vi "PH_IEEE1394Camera.set Cam Attribute GUI Elements for the first Time.vi"(0 "i ref in":refnum<vi>, 5 "error in (no error)":errorcluster) -> (14 "i ref out":refnum<vi>, 19 "error out":errorcluster)   [LabVIEW 2014, in "PH_IEEE1394Camera.lvlib"]
doc: "This VI gets several cam trigger attributes, sets them to own attributes and the GUI elements."
uses:
  PH_IEEE1394Camera.lvlib
  PH_Basics/PH_Common/PH_Common.lvlib
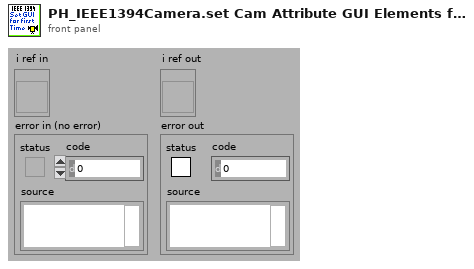
[diagram p1: front panel]
types:
  T1 = typedef "PH_IEEE1394Camera.lvlib/PH_IEEE1394Camera.i attribute.ctl" = cluster{"Gui Refs":cluster{"Brightness":refnum<vi>, "Shutter":refnum<vi>, "Gain":refnum<vi>, "Center of Gravity":refnum<vi>, "Supported Video Modes":refnum<vi>, "Trigger Polarity":refnum<vi>, "Trigger Mode":refnum<vi>, "Trigger Timeout":refnum<vi>, "Bit Depth":refnum<vi>, "Video Mode":refnum<vi>, "Top":refnum<vi>, "Bottom":refnum<vi>, "Left":refnum<vi>, "Right":refnum<vi>, "Set ROI to Maximum":refnum<vi>, "Camera Details":refnum<vi>, "Current Cam Attributes":refnum<vi>, "Attribute to set":refnum<vi>, "Num Value":refnum<vi>, "String Value":refnum<vi>, "Bool Value":refnum<vi>, "Set Cam Attribute":refnum<vi>}, "Cam":cluster{"IMAQ1394 Session":T2, "Camera Details":T3}, "Current Attributes":T4[], "Supported Video Modes ":cluster{"Video Mode":u32, "Video Mode Name":string}[], "Wanted Attributes":cluster{"Name":string, "Num Value":dbl, "String Value":string, "Boolean Value":bool}[], "Cam Attributes":T6}
  T2 = typedef "IMAQdx.ctl" = refnum<k21>
  T3 = typedef "PH_IEEE1394Camera.lvlib/PH_IEEE1394Camera.Cam Details.ctl" = cluster{"Model":string, "Serial Number":dbl, "Cam name (Machinery)":string, "Bus Type":string}
  T4 = typedef "PH_IEEE1394Camera.lvlib/PH_IEEE1394Camera.Cam Attribute.ctl" = cluster{"Information":cluster{"Type":T5, "Readable":bool, "Writable":bool, "Name":string}, "Num Value":dbl, "String Value":string, "Maximum":dbl, "Minimum":dbl, "Units":string, "Description":string, "EnumStrings[]":string[], "EnumValues[]":u32[], "Boolean Value":bool}
  T5 = typedef "NI_Vision_Acquisition_Software.lvlib/IMAQdx Attribute Type.ctl" = enum32{"U32", "I64", "DBL", "String", "Enum", "Bool", "Command"}
  T6 = typedef "PH_IEEE1394Camera.lvlib/PH_IEEE1394Camera.Relevant Cam Attributes.ctl" = cluster{"Video Mode":cluster{"Name":string, "Index":i32}, "Brightness":cluster{"Name":string, "Index":i32}, "Gain":cluster{"Name":string, "Index":i32}, "Shutter":cluster{"Name":string, "Index":i32}, "Trigger Pol":cluster{"Name":string, "Index":i32}, "Trigger Mode":cluster{"Name":string, "Index":i32}, "Timeout":cluster{"Name":string, "Index":i32}, "Bit Depth":cluster{"Name":string, "Index":i32}, "Pixel Bits":cluster{"Name":string, "Index":i32}, "Pixel Bytes":cluster{"Name":string, "Index":i32}, "Left":cluster{"Name":string, "Index":i32}, "Right":cluster{"Name":string, "Index":i32}, "Top":cluster{"Name":string, "Index":i32}, "Bottom":cluster{"Name":string, "Index":i32}}
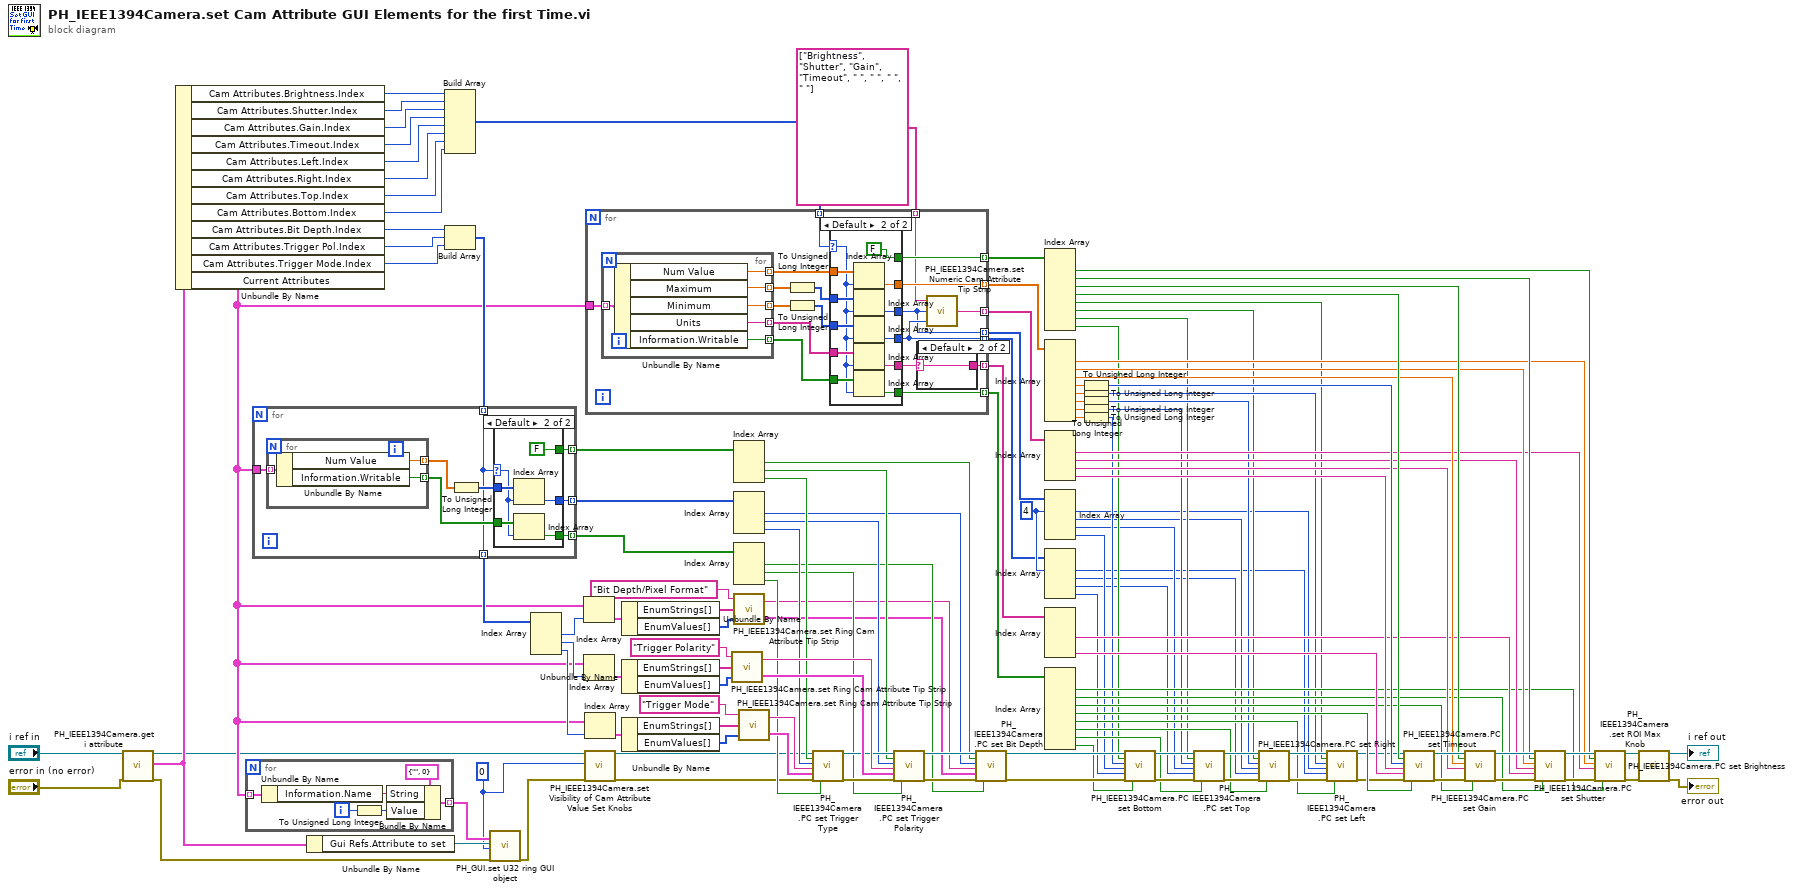
[diagram p0: block diagram]
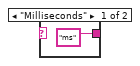
[diagram p2: hidden frame]
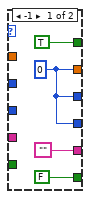
[diagram p3: hidden frame]
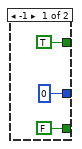
[diagram p4: hidden frame]
diagram:
  w1 = u32 0 ("Value")
  w25 = 4 ("index")
  n1 = call "PH_IEEE1394Camera.get i attribute.vi"("i ref in"="i ref in", "error in (no error)"="error in (no error)") -> ("i ref out"=w5:refnum<vi>, "i attribute"=w7:T1, "error out"=w8:errorcluster)  [unwired: 15 in]
  n2 = Unbundle By Name(w7) -> ("Cam Attributes.Brightness.Index"=w91:i32, "Cam Attributes.Shutter.Index"=w90:i32, "Cam Attributes.Gain.Index"=w89:i32, "Cam Attributes.Timeout.Index"=w88:i32, "Cam Attributes.Left.Index"=w55:i32, "Cam Attributes.Right.Index"=w54:i32, "Cam Attributes.Top.Index"=w53:i32, "Cam Attributes.Bottom.Index"=w52:i32, "Cam Attributes.Bit Depth.Index"=w133:i32, "Cam Attributes.Trigger Pol.Index"=w128:i32, "Cam Attributes.Trigger Mode.Index"=w127:i32, "Current Attributes"=w10:T4[])
  n3 = for {
    tunnel: w10 -> [w141] mode=indexing
    tunnel: [w138] -> w9 mode=indexing
    i -> [w137]
    n4 = Unbundle By Name(w141) -> ("Information.Name"=w139:string)
    n5 = To Unsigned Long Integer(number=w137) -> (unsigned 32bit integer=w136:u32)
    n6 = Bundle By Name(cluster=cluster{"String":string, "Value":u32} {"String"="", "Value"=0}, "String"=w139, "Value"=w136) -> (w138:cluster{"String":string, "Value":u32})
  }
  n7 = Unbundle By Name(w7) -> ("Gui Refs.Attribute to set"=w6:refnum<vi>)
  n8 = Build Array(w91, w90, w89, w88, w55, w54, w53, w52) -> (w87:i32[])
  n9 = Build Array(w133, w128, w127) -> (w132:i32[])
  n10 = for {
    tunnel: w10 -> [w149]
    tunnel: w132 -> [w142] mode=indexing
    tunnel: [w145] -> w130 mode=indexing
    tunnel: [w144] -> w129 mode=indexing
    tunnel: [w143] -> w131 mode=indexing
    tunnel: [w142] -> w112 mode=indexing
    n11 = for {
      tunnel: w149 -> [w161] mode=indexing
      tunnel: [w160] -> w148 mode=indexing
      tunnel: [w159] -> w146 mode=indexing
      n12 = Unbundle By Name(w161) -> ("Num Value"=w160:dbl, "Information.Writable"=w159:bool)
    }
    n13 = To Unsigned Long Integer(number=w148) -> (unsigned 32bit integer=w147:u32[])
    n14 = case shown="Default" w142 {
      selector: w142 -> [_ w153]
      tunnel: w147 -> [_ w158]
      tunnel: w146 -> [_ w157]
      tunnel: [u32 0 ("Num Value") w156] -> w145
      tunnel: [FALSE ("Writable") w155] -> w144
      tunnel: [TRUE ("Writable") FALSE ("Writable")] -> w143
      frame -1 {
      }
      frame Default {
        n15 = Index Array(array=w158, index=w153) -> (element=w156:u32)
        n16 = Index Array(array=w157, index=w153) -> (element=w155:bool)
      }
    }
  }
  n17 = call "PH_GUI.set U32 ring GUI object.vi"("Strings And Values [Empty]"=w9, "Ring Ref"=w6, "Value"=w1, "error in (no error)"=w8) -> ("error out"=w3:errorcluster)  [unwired: 15 in]
  n18 = Index Array(array=w112) -> (element #1=w97:i32, element #2=w111:i32, element #3=w110:i32)  [unwired: 3 in]
  n19 = Index Array(array=w10, index=w97) -> (element=w98:T4)
  n20 = Index Array(array=w10, index=w111) -> (element=w109:T4)
  n21 = Index Array(array=w10, index=w110) -> (element=w108:T4)
  n22 = call "PH_IEEE1394Camera.set Visibility of Cam Attribute Value Set Knobs.vi"("VI in"=w5, "Index of selected Attribute"=w1, "error in (no error)"=w3) -> ("VI out"=w4:refnum<vi>, "error out"=w2:errorcluster)  [unwired: 15 in]
  n23 = for {
    tunnel: w10 -> [w179]
    tunnel: w87 -> [w162] mode=indexing
    tunnel: [w172] -> w74 mode=indexing
    tunnel: [w168] -> w63 mode=indexing
    tunnel: [w171] -> w60 mode=indexing
    tunnel: [w170] -> w82 mode=indexing
    tunnel: string[] ["Brightness", "Shutter", "Gain", "Timeout", " ", " ", " ", " "] -> [w167] mode=indexing
    tunnel: [w166] -> w68 mode=indexing
    tunnel: [w164] -> w23 mode=indexing
    tunnel: [w163] -> w24 mode=indexing
    n24 = for {
      tunnel: w179 -> [w203] mode=indexing
      tunnel: [w202] -> w165 mode=indexing
      tunnel: [w201] -> w178 mode=indexing
      tunnel: [w200] -> w177 mode=indexing
      tunnel: [w199] -> w174 mode=indexing
      tunnel: [w198] -> w173 mode=indexing
      n25 = Unbundle By Name(w203) -> ("Num Value"=w202:dbl, "Maximum"=w201:dbl, "Minimum"=w200:dbl, "Units"=w199:string, "Information.Writable"=w198:bool)
    }
    n26 = To Unsigned Long Integer(number=w178) -> (unsigned 32bit integer=w176:u32[])
    n27 = To Unsigned Long Integer(number=w177) -> (unsigned 32bit integer=w175:u32[])
    n28 = case shown="Default" w162 {
      selector: w162 -> [_ w186]
      tunnel: w165 -> [_ w197]
      tunnel: w176 -> [_ w196]
      tunnel: w175 -> [_ w195]
      tunnel: w174 -> [_ w194]
      tunnel: w173 -> [_ w193]
      tunnel: [w185 w192] -> w172
      tunnel: [w185 w191] -> w163
      tunnel: [w185 w190] -> w164
      tunnel: ["" w189] -> w169
      tunnel: [FALSE ("Writable") w188] -> w171
      tunnel: [TRUE ("Writable") FALSE ("Writable")] -> w170
      frame -1 {
        w185 = u32 0 ("Num Value")
      }
      frame Default {
        n29 = Index Array(array=w197, index=w186) -> (element=w192:dbl)
        n30 = Index Array(array=w196, index=w186) -> (element=w191:u32)
        n31 = Index Array(array=w195, index=w186) -> (element=w190:u32)
        n32 = Index Array(array=w194, index=w186) -> (element=w189:string)
        n33 = Index Array(array=w193, index=w186) -> (element=w188:bool)
      }
    }
    n34 = case shown="Default" w169 {
      selector: w169 -> [_ w181]
      tunnel: ["ms" w181] -> w168
      frame "Milliseconds" {
      }
      frame Default {
      }
    }
    n35 = call "PH_IEEE1394Camera.set Numeric Cam Attribute Tip Strip.vi"("Minimum"=w164, "Maximum"=w163, "Attribute"=w167) -> ("Tip Strip"=w166:string)
  }
  n36 = Unbundle By Name(w98) -> ("EnumStrings[]"=w95:string[], "EnumValues[]"=w96:u32[])
  n37 = Unbundle By Name(w109) -> ("EnumStrings[]"=w104:string[], "EnumValues[]"=w105:u32[])
  n38 = Unbundle By Name(w108) -> ("EnumStrings[]"=w107:string[], "EnumValues[]"=w106:u32[])
  n39 = call "PH_IEEE1394Camera.set Ring Cam Attribute Tip Strip.vi"("EnumValues[]"=w105, "EnumStrings[]"=w104, "Attribute Name"="Trigger Polarity") -> ("Strings and Values"=w126:cluster{"String":string, "Value":u32}[], "Tip Strip"=w125:string)
  n40 = Index Array(array=w131) -> (element #1=w100:bool, element #2=w120:bool, element #3=w119:bool)  [unwired: 3 in]
  n41 = Index Array(array=w130) -> (element #1=w99:u32, element #2=w118:u32, element #3=w117:u32)  [unwired: 3 in]
  n42 = Index Array(array=w129) -> (element #1=w101:bool, element #2=w116:bool, element #3=w115:bool)  [unwired: 3 in]
  n43 = call "PH_IEEE1394Camera.set Ring Cam Attribute Tip Strip.vi"("EnumValues[]"=w96, "EnumStrings[]"=w95, "Attribute Name"="Bit Depth/Pixel Format") -> ("Strings and Values"=w93:cluster{"String":string, "Value":u32}[], "Tip Strip"=w92:string)
  n44 = call "PH_IEEE1394Camera.set Ring Cam Attribute Tip Strip.vi"("EnumValues[]"=w106, "EnumStrings[]"=w107, "Attribute Name"="Trigger Mode") -> ("Strings and Values"=w124:cluster{"String":string, "Value":u32}[], "Tip Strip"=w123:string)
  n45 = call "PH_IEEE1394Camera.PC set Trigger Type.vi"("i ref in"=w4, "No Info? (False)"=w119, "Trigger Mode"=w117, "Tip Strip [Empty]"=w123, "Strings And Values [Empty]"=w124, "error in (no error)"=w2, "Trigger Mode writable? (True)"=w115) -> ("i ref out"=w122:refnum<vi>, "error out"=w121:errorcluster)  [unwired: 11 in]
  n46 = call "PH_IEEE1394Camera.PC set Trigger Polarity.vi"("i ref in"=w122, "No Info? (False)"=w120, "Trigger Polarity"=w118, "Tip Strip [Empty]"=w125, "Strings And Values [Empty]"=w126, "error in (no error)"=w121, "Trigger Polarity writable? (True)"=w116) -> ("i ref out"=w103:refnum<vi>, "error out"=w102:errorcluster)  [unwired: 11 in]
  n47 = call "PH_IEEE1394Camera.PC set Bit Depth.vi"("i ref in"=w103, "No Info? (False)"=w100, "Bit Depth"=w99, "Tip Strip [Empty]"=w92, "Strings And Values [Empty]"=w93, "error in (no error)"=w102, "Bit Depth writable? (True)"=w101) -> ("i ref out"=w46:refnum<vi>, "error out"=w48:errorcluster)  [unwired: 11 in]
  n48 = Index Array(array=w82) -> (element #1=w78:bool, element #2=w77:bool, element #3=w76:bool, element #4=w75:bool, element #5=w26:bool, element #6=w27:bool, element #7=w28:bool, element #8=w29:bool)  [unwired: 8 in]
  n49 = Index Array(array=w74) -> (element #1=w73:dbl, element #2=w72:dbl, element #3=w71:dbl, element #4=w70:dbl, element #5=w34:dbl, element #6=w35:dbl, element #7=w36:dbl, element #8=w37:dbl)  [unwired: 8 in]
  n50 = Index Array(array=w68) -> (element #1=w67:string, element #2=w66:string, element #3=w65:string, element #4=w64:string)  [unwired: 4 in]
  n51 = Index Array(array=w24, index #1=w25) -> (element #1=w22:u32, element #2=w21:u32, element #3=w20:u32, element #4=w19:u32)  [unwired: 3 in]
  n52 = Index Array(array=w23, index #1=w25) -> (element #1=w15:u32, element #2=w16:u32, element #3=w17:u32, element #4=w18:u32)  [unwired: 3 in]
  n53 = Index Array(array=w63) -> (element #2=w61:string, element #4=w62:string)  [unwired: 4 in, 2 out]
  n54 = Index Array(array=w60) -> (element #1=w59:bool, element #2=w58:bool, element #3=w57:bool, element #4=w56:bool, element #5=w38:bool, element #6=w39:bool, element #7=w40:bool, element #8=w41:bool)  [unwired: 8 in]
  n55 = To Unsigned Long Integer(number=w70) -> (unsigned 32bit integer=w69:u32)
  n56 = To Unsigned Long Integer(number=w34) -> (unsigned 32bit integer=w30:u32)
  n57 = To Unsigned Long Integer(number=w35) -> (unsigned 32bit integer=w31:u32)
  n58 = To Unsigned Long Integer(number=w36) -> (unsigned 32bit integer=w32:u32)
  n59 = To Unsigned Long Integer(number=w37) -> (unsigned 32bit integer=w33:u32)
  n60 = call "PH_IEEE1394Camera.PC set Bottom.vi"("i ref in"=w46, "No Info? (False)"=w29, "Bottom"=w33, "Maximum Bottom"=w19, "Minimum Bottom"=w18, "error in (no error)"=w48, "Bottom writable? (True)"=w41) -> ("i ref out"=w45:refnum<vi>, "error out"=w51:errorcluster)  [unwired: 11 in]
  n61 = call "PH_IEEE1394Camera.PC set Top.vi"("i ref in"=w45, "No Info? (False)"=w28, "Top"=w32, "Maximum Top"=w20, "Minimum Top"=w17, "error in (no error)"=w51, "Top writable? (True)"=w40) -> ("i ref out"=w44:refnum<vi>, "error out"=w50:errorcluster)  [unwired: 11 in]
  n62 = call "PH_IEEE1394Camera.PC set Right.vi"("i ref in"=w44, "No Info? (False)"=w27, "Right"=w31, "Maximum Right"=w21, "Minimum Right"=w16, "error in (no error)"=w50, "Right writable? (True)"=w39) -> ("i ref out"=w43:refnum<vi>, "error out"=w49:errorcluster)  [unwired: 11 in]
  n63 = call "PH_IEEE1394Camera.PC set Left.vi"("i ref in"=w43, "No Info? (False)"=w26, "Left"=w30, "Maximum Left"=w22, "Minimum Left"=w15, "error in (no error)"=w49, "Left writable? (True)"=w38) -> ("i ref out"=w42:refnum<vi>, "error out"=w47:errorcluster)  [unwired: 11 in]
  n64 = call "PH_IEEE1394Camera.PC set Timeout.vi"("i ref in"=w42, "No Info? (False)"=w75, "Timeout"=w69, "Tip Strip"=w64, "Unit"=w62, "error in (no error)"=w47, "Timeout writable? (True)"=w56) -> ("i ref out"=w85:refnum<vi>, "error out"=w81:errorcluster)  [unwired: 11 in]
  n65 = call "PH_IEEE1394Camera.PC set Gain.vi"("i ref in"=w85, "No Info? (False)"=w76, "Gain"=w71, "Tip Strip"=w65, "error in (no error)"=w81, "Gain writable? (True)"=w57) -> ("i ref out"=w84:refnum<vi>, "error out"=w80:errorcluster)  [unwired: 12 in]
  n66 = call "PH_IEEE1394Camera.PC set Shutter.vi"("i ref in"=w84, "No Info? (False)"=w77, "Shutter"=w72, "Tip Strip"=w66, "Unit"=w61, "error in (no error)"=w80, "Shutter writable? (True)"=w58) -> ("i ref out"=w83:refnum<vi>, "error out"=w79:errorcluster)  [unwired: 11 in]
  n67 = call "PH_IEEE1394Camera.PC set Brightness.vi"("i ref in"=w83, "No Info? (False)"=w78, "Brightness"=w73, "Tip Strip"=w67, "error in (no error)"=w79, "Brightness writable? (True)"=w59) -> ("i ref out"=w13:refnum<vi>, "error out"=w14:errorcluster)  [unwired: 12 in]
  n68 = call "PH_IEEE1394Camera.set ROI Max Knob.vi"("VI in"=w13, "error in (no error)"=w14) -> ("VI out"=→"i ref out":refnum<vi>, "error out"=→"error out":errorcluster)  [unwired: 16 in]
